vi "Read Input Registers.vi"(7 "unit ID":u8, 8 "error in":errorcluster, 9 "number of inputs":u16, 10 "starting address":u16, 11 "Modbus master in":refnum<class "Modbus Master.lvclass">) -> (0 "error out":errorcluster, 2 "register values":u16[](array[numeric]), 3 "Modbus master out":refnum<class "Modbus Master.lvclass">)   [LabVIEW 2013, in "Modbus Library - Advance.lvlib" / "Modbus Master.lvclass"]
doc: "Reads <B>number of inputs</B> input registers starting at <B>starting address</B> from the device."
uses:
  Modbus Master.lvclass
  Modbus Master.lvclass/Modbus Master.ctl
  Modbus API.lvclass/Modbus API.ctl
  Transmission Data Unit/Transmission Data Unit.lvclass/Transmission Data Unit.ctl
  Transmission Data Unit/Transmission Data Unit.lvclass
  Modbus API.lvclass
  Master Function Definition/Master Function Definition.lvclass
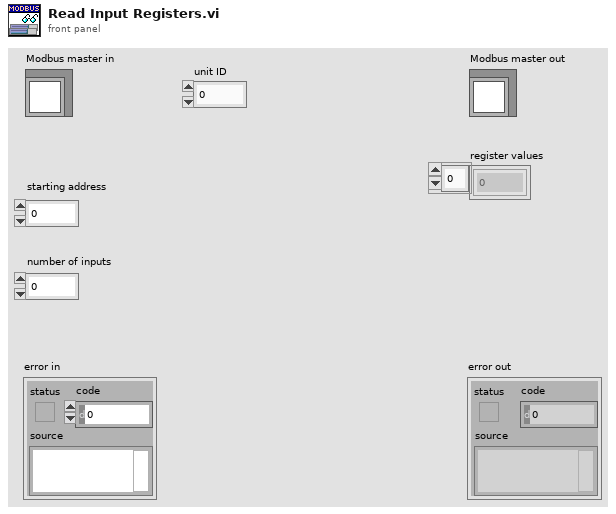
[diagram p1: front panel]
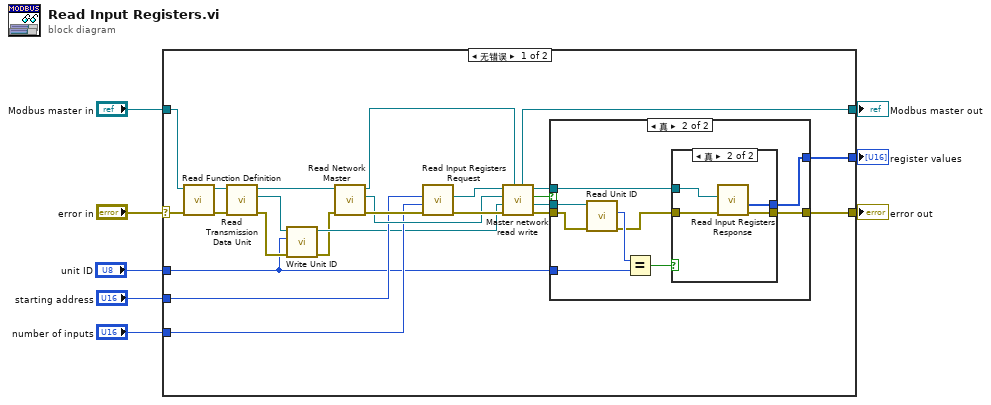
[diagram p0: block diagram]
diagram:
  n1 = case shown="无错误" "error in" {
    selector: "error in" -> [w24 w49]
    tunnel: [w25 w49] -> w7
    tunnel: [w19 w48] -> w6
    tunnel: "Modbus master in" -> [w18 w48]
    tunnel: [w20 _] -> w4
    tunnel: "starting address" -> [w17 _]
    tunnel: "number of inputs" -> [w16 _]
    tunnel: "unit ID" -> [w9 _]
    frame No Error {
      n2 = call "Read Function Definition.vi"("error in"=w24, "Modbus master in"=w18) -> ("error out"=w31:errorcluster, "Modbus master out"=w32:refnum<class "Modbus Master.lvclass">)  [unwired: 7 in, 1 out]
      n3 = call "Read Transmission Data Unit.vi"("error in"=w31, "Modbus instance in"=w32) -> ("error out"=w12:errorcluster, "transmission data unit"=w14:refnum<class "Transmission Data Unit.lvclass">, "Modbus instance out"=w30:refnum<class "Modbus Master.lvclass">)  [unwired: 7 in]
      n4 = call "Write Unit ID.vi"("error in"=w12, "unit ID"=w9, "transmission data unit in"=w14) -> ("error out"=w11:errorcluster, "transmission data unit out"=w13:refnum<class "Transmission Data Unit.lvclass">)  [unwired: 7 in]
      n5 = call "Read Network Master.vi"("error in"=w11, "Modbus master in"=w30) -> ("error out"=w26:errorcluster, "network master"=w21:refnum<class "Network Master.lvclass">, "Modbus master out"=w27:refnum<class "Modbus Master.lvclass">)  [unwired: 7 in]
      n6 = call "Read Input Registers Request.vi"("error in"=w26, "Number of Registers"=w16, "Starting Address"=w17) -> ("error out"=w28:errorcluster, "modbus data unit out"=w22:refnum<class "Modbus Data Unit.lvclass">)  [unwired: 7 in]
      n7 = call "Master network read write.vi"("Modbus master in"=w27, "error in"=w28, "transmission data unit in"=w13, "network master in"=w21, "Modbus data unit in"=w22) -> ("error out"=w29:errorcluster, "transmission data unit out"=w10:refnum<class "Transmission Data Unit.lvclass">, "PDU Valid?"=w15:bool, "Modbus data unit out"=w23:refnum<class "Modbus Data Unit.lvclass">, "Modbus master out"=w19:refnum<class "Modbus Master.lvclass">)  [unwired: 2 in]
      n8 = case shown="真" w15 {
        tunnel: w29 -> [w33 w38]
        tunnel: [w33 w42] -> w25
        tunnel: w23 -> [_ w41]
        tunnel: [_ w40] -> w20
        tunnel: w10 -> [_ w39]
        tunnel: w9 -> [_ w36]
        frame False {
        }
        frame True {
          n9 = call "Read Unit ID.vi"("error in"=w38, "transmission data unit in"=w39) -> ("error out"=w35:errorcluster, "unit ID"=w37:u8)  [unwired: 7 in, 1 out]
          n10 = Equal?(x=w37, y=w36) -> (x = y?=w34:bool)
          n11 = case shown="真" w34 {
            tunnel: [w43 w47] -> w42
            tunnel: w41 -> [_ w46]
            tunnel: [_ w45] -> w40
            tunnel: w35 -> [w43 w44]
            frame False {
            }
            frame True {
              n12 = call "Read Input Registers Response.vi"("error in"=w44, "modbus data unit in"=w46) -> ("error out"=w47:errorcluster, "Register Values"=w45:u16[])  [unwired: 7 in, 1 out]
            }
          }
        }
      }
    }
    frame Error {
    }
  }
  "error out" <- w7
  "Modbus master out" <- w6
  "register values" <- w4
